vi "Josey Random Variables.vi"() -> ()   [LabVIEW 2010]
uses:
  <vilib>/Utility/file.llb/Write To Spreadsheet File (DBL).vi
  <vilib>/Analysis/NI_AALBase.lvlib
panel:
  in  "file path (dialog if empty)":path
  out "Histogram":T1(graph)
  in  "Hitogram Interval":i32
  out "Waveform Graph or Random Numbers":dbl[](graph)
  in  "Desired Expected Random Number":dbl
  in  "Number of Random #'s":i32
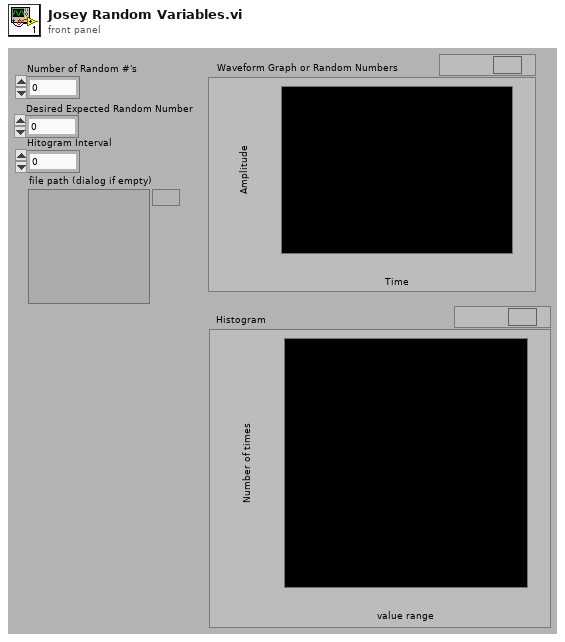
[diagram p1: front panel]
types:
  T1 = cluster{"X Values":dbl[], "Histogram: h(x)":i32[]}
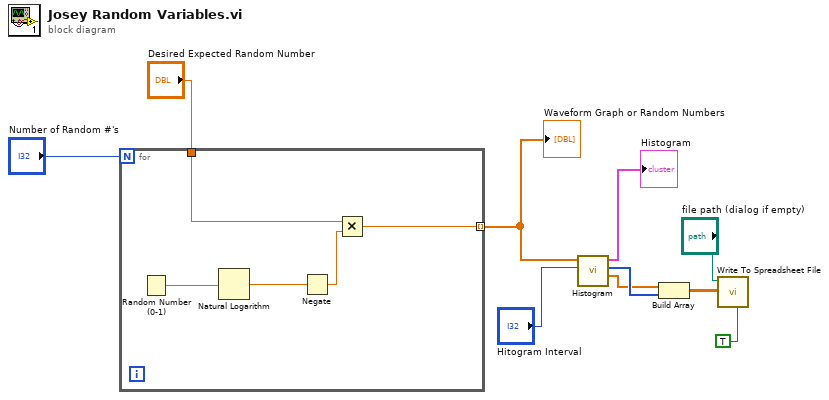
[diagram p0: block diagram]
diagram:
  n1 = for {
    N: "Number of Random #'s" -> [_]
    tunnel: "Desired Expected Random Number" -> [w15]
    tunnel: [w11] -> w8 mode=indexing
    n2 = Random Number (0-1)() -> (number: 0 to 1=w14:dbl)
    n3 = Natural Logarithm(1:w14) -> (0:w13:dbl)
    n4 = Negate(x=w13) -> (-x=w12:dbl)
    n5 = Multiply(x=w15, y=w12) -> (x*y=w11:dbl)
  }
  "Waveform Graph or Random Numbers" <- w8
  n6 = call <vilib>:"Histogram.vi"("intervals"="Hitogram Interval", "X"=w8) -> ("X Values"=w4:dbl[], "Histogram: h(x)"=w5:i32[], "Histogram Graph"=→"Histogram":T1)  [unwired: 6 in, 1 out]
  n7 = Build Array(w4, w5) -> (w3:dbl[][])
  n8 = call-poly <vilib>:"Write To Spreadsheet File.vi"("transpose? (no:F)"=TRUE, "2D data"=w3, "file path (dialog if empty)"="file path (dialog if empty)") -> ()  [unwired: 5 in, 1 out]
